vi "Test Initialize Scarce.vi"(8 "error in":errorcluster) -> (0 "error out":errorcluster)   [LabVIEW 2020]
uses:
  <vilib>/addons/_JKI Toolkits/Caraya/classes/Test/Test.lvclass
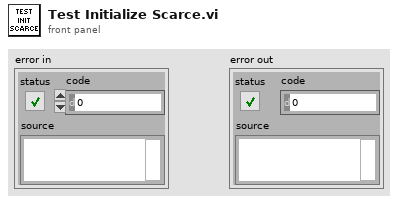
[diagram p1: front panel]
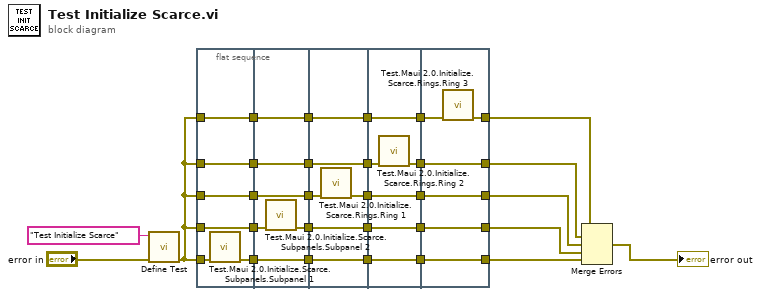
[diagram p0: block diagram]
diagram:
  n1 = call <vilib>:"Define Test.vi"("error in (no error)"="error in", "Label (VI Title)"="Test Initialize Scarce") -> ("error out"=w6:errorcluster)  [unwired: 9 in]
  n2 = flat-sequence {
    tunnel: w6 -> [w35]
    tunnel: [w35] -> w27
    tunnel: w6 -> [w34]
    tunnel: [w34] -> w26
    tunnel: w6 -> [w33]
    tunnel: [w33] -> w25
    tunnel: [w32] -> w16
    tunnel: w6 -> [w31]
    tunnel: w6 -> [w30]
    tunnel: [w30] -> w5
    tunnel: w27 -> [w38]
    tunnel: w26 -> [w41]
    tunnel: [w41] -> w24
    tunnel: w25 -> [w40]
    tunnel: [w40] -> w23
    tunnel: [w37] -> w22
    tunnel: [w39] -> w21
    tunnel: w16 -> [w39]
    tunnel: w5 -> [w36]
    tunnel: [w36] -> w4
    tunnel: w24 -> [w44]
    tunnel: w23 -> [w47]
    tunnel: [w47] -> w20
    tunnel: [w43] -> w19
    tunnel: [w46] -> w18
    tunnel: w22 -> [w46]
    tunnel: [w45] -> w17
    tunnel: w21 -> [w45]
    tunnel: w4 -> [w42]
    tunnel: [w42] -> w3
    tunnel: w20 -> [w49]
    tunnel: w19 -> [w53]
    tunnel: w18 -> [w52]
    tunnel: w17 -> [w51]
    tunnel: [w53] -> w10
    tunnel: [w52] -> w9
    tunnel: [w51] -> w8
    tunnel: [w50] -> w7
    tunnel: w3 -> [w48]
    tunnel: [w48] -> w2
    tunnel: [w56] -> w14
    tunnel: [w57] -> w11
    tunnel: [w58] -> w12
    tunnel: [w59] -> w13
    tunnel: w10 -> [w59]
    tunnel: w9 -> [w58]
    tunnel: w8 -> [w57]
    tunnel: w7 -> [w56]
    tunnel: w2 -> [w55]
    tunnel: [w54] -> w1
    frame #0 {
      n3 = call "Test.Maui 2.0.Initialize.Scarce.Subpanels.Subpanel 1.vi"("error in"=w31) -> ("error out"=w32:errorcluster)  [unwired: 10 in]
    }
    frame #1 {
      n4 = call "Test.Maui 2.0.Initialize.Scarce.Subpanels.Subpanel 2.vi"("error in"=w38) -> ("error out"=w37:errorcluster)  [unwired: 10 in]
    }
    frame #2 {
      n5 = call "Test.Maui 2.0.Initialize.Scarce.Rings.Ring 1.vi"("error in"=w44) -> ("error out"=w43:errorcluster)  [unwired: 10 in]
    }
    frame #3 {
      n6 = call "Test.Maui 2.0.Initialize.Scarce.Rings.Ring 2.vi"("error in"=w49) -> ("error out"=w50:errorcluster)  [unwired: 10 in]
    }
    frame #4 {
      n7 = call "Test.Maui 2.0.Initialize.Scarce.Rings.Ring 3.vi"("error in"=w55) -> ("error out"=w54:errorcluster)  [unwired: 10 in]
    }
  }
  n8 = Merge Errors(w1, w14, w13, w12, w11) -> (→"error out":errorcluster)
